vi "IVA_Adjust_Dynamic.vi"(8 "error in (no error)":errorcluster, 10 "Image Type":T1 items=["Grayscale (U8)", "Grayscale (I16)", "Grayscale (SGL)", "Complex (CSG)", "RGB (U32)", "HSL (U32)", "RGB (U64)", "Grayscale (U16)"], 11 "Image Src":T2) -> (0 "error out":errorcluster, 3 "Image Out":T2)   [LabVIEW 2017]
uses:
  <vilib>/vision/Image Controls.llb/IMAQ Image.ctl
  <vilib>/vision/NI_Vision_Development_Module.lvlib
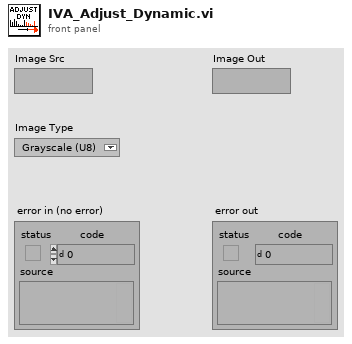
[diagram p1: front panel]
types:
  T1 = typedef "Image Type" = u32
  T2 = typedef "IMAQ Image.ctl" = refnum<image>
  T3 = cluster{"histogram":u32[], "Minimal Value":sgl, "Maximal Value":sgl, "Starting Value":sgl, "Interval Width":sgl, "Mean Value":sgl, "Standard  Variation":sgl, "Area (pixels)":i32}
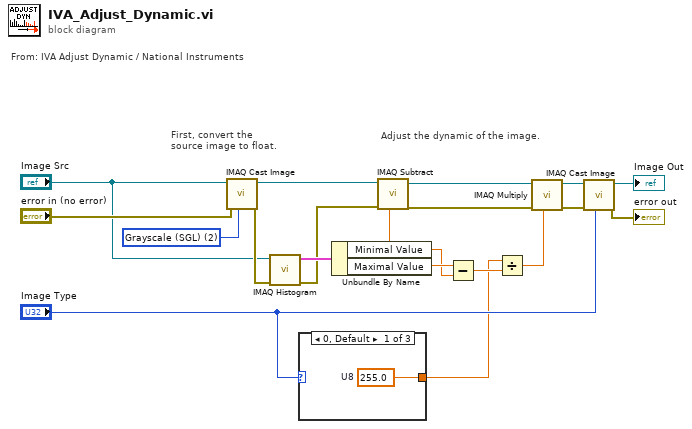
[diagram p0: block diagram]
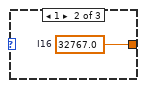
[diagram p2: hidden frame]
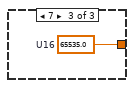
[diagram p3: hidden frame]
diagram:
  w19 = T1 2 items=["Grayscale (U8)", "Grayscale (I16)", "Grayscale (SGL)", "Complex (CSG)", "RGB (U32)", "HSL (U32)", "RGB (U64)", "Grayscale (U16)"] ("Image Type")
  # "From: IVA Adjust Dynamic / National Instruments"
  # "Adjust the dynamic of the image."
  # "First, convert the\nsource image to float."
  n1 = call "IMAQ Cast Image"("Image Type"=w19, "error in (no error)"="error in (no error)", "Image Src"="Image Src") -> ("error out"=w12:errorcluster, "Image Dst Out"=w13:T2)  [unwired: 3 in, 4 out]
  n2 = call "IMAQ Histogram"("error in (no error)"=w12, "Image"="Image Src") -> ("error out"=w8:errorcluster, "Histogram Report"=w17:T3)  [unwired: 3 in, 5 out]
  n3 = case shown="0, Default" "Image Type" {
    tunnel: [w20 w21 w22] -> w1
    frame 0, Default {
      w20 = sgl 255.0  # U8
    }
    frame 1 {
      w21 = sgl 32767.0  # I16
    }
    frame 7 {
      w22 = sgl 65535.0  # U16
    }
  }
  n4 = Unbundle By Name(w17) -> ("Minimal Value"=w10:sgl, "Maximal Value"=w16:sgl)
  n5 = call "IMAQ Subtract"("Image Src A"=w13, "Constant"=w10, "error in (no error)"=w8) -> ("Image Dst Out"=w14:T2, "error out"=w7:errorcluster)  [unwired: 2 in, 2 out]
  n6 = Subtract(x=w16, y=w10) -> (x-y=w15:sgl)
  n7 = Divide(x=w1, y=w15) -> (x/y=w9:sgl)
  n8 = call "IMAQ Multiply"("Image Src A"=w14, "Constant"=w9, "error in (no error)"=w7) -> ("Image Dst Out"=w6:T2, "error out"=w5:errorcluster)  [unwired: 2 in, 2 out]
  n9 = call "IMAQ Cast Image"("Image Type"="Image Type", "error in (no error)"=w5, "Image Src"=w6) -> ("error out"=→"error out":errorcluster, "Image Dst Out"=→"Image Out":T2)  [unwired: 3 in, 4 out]
